vi "MDPtr To FlattenStrPtr.vi"(1 "HexStrPtr":T1) -> (0 "FlattenStrPtr":string)   [LabVIEW 2017, in "MDPtr.lvlib"]
uses:
  MDPtr.lvlib
  MDPtr TypeDef/MDPtr.ctl
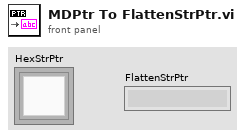
[diagram p1: front panel]
types:
  T1 = typedef "MDPtr.lvlib/MDPtr.ctl" = refnum<k1>
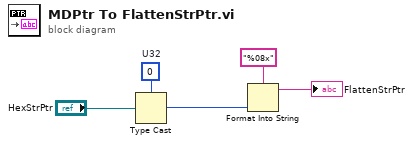
[diagram p0: block diagram]
diagram:
  w3 = 0  # U32
  n1 = Type Cast(type=w3, x="HexStrPtr") -> (*(type *) &x=w2:i32)
  n2 = Format Into String(format string="%08x", w2) -> (resulting string=→"FlattenStrPtr":string)  [unwired: 2 in, 1 out]
